vi "UI Initialize.vi"(8 "error in (no error)":errorcluster, 11 "TestEngine in":refnum<class "TestEngine.lvclass">) -> (0 "error out":errorcluster, 3 "TestEngine out":refnum<class "TestEngine.lvclass">)   [LabVIEW 2019, in "TestEngine.lvlib" / "TestEngine.lvclass"]
uses:
  TestEngine.lvclass
  C:/Program Files (x86)/National Instruments/LabVIEW 2019/vi.lib/NI/Event Source Actor/Event Source/Event Source/Event Source.lvclass
  TestEngineReference.lvclass
  C:/Program Files (x86)/National Instruments/LabVIEW 2019/vi.lib/NI/Event Source Actor/Event Source/Event/Event.lvclass
  <vilib>/NI/Event Source Actor/Event Source/Event/Event.lvclass/Event.ctl
  TestEngine.lvclass/TestEngine.ctl
  <vilib>/NI/Event Source Actor/Event Source/Event/Event.lvclass
  <vilib>/NI/Event Source Actor/Event Source/Event Source/Event Source.lvclass
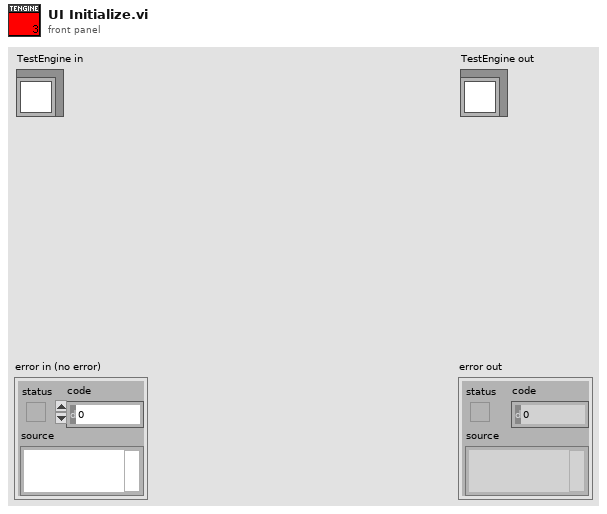
[diagram p1: front panel]
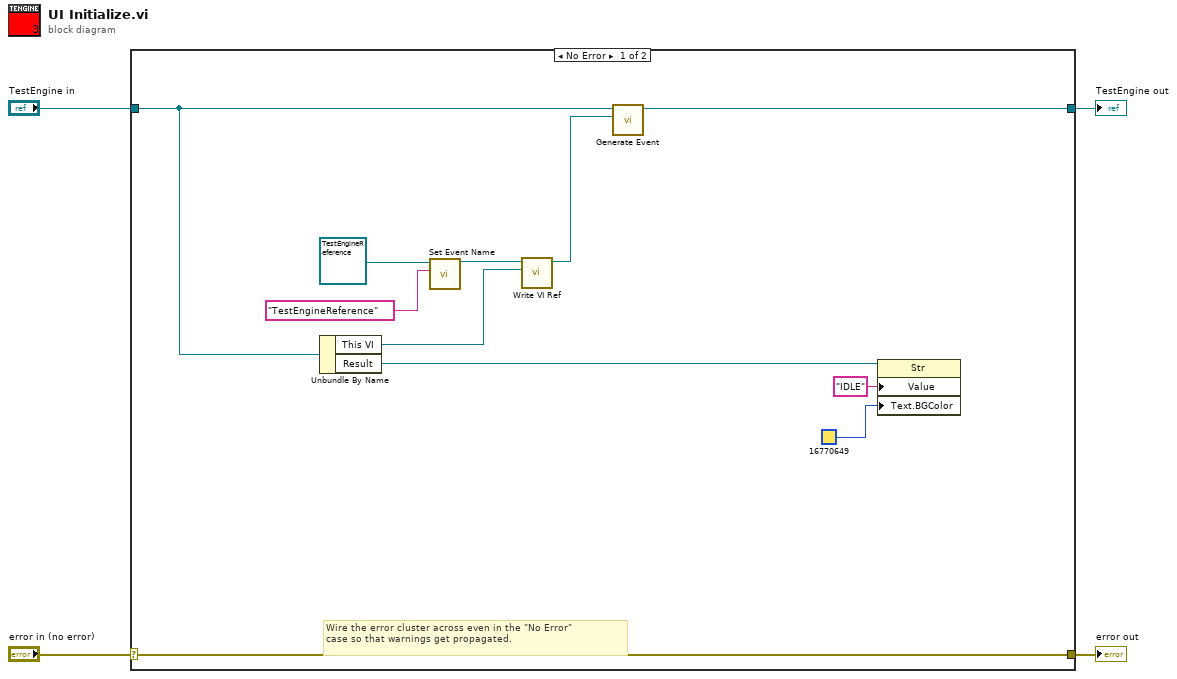
[diagram p0: block diagram]
diagram:
  n1 = case shown="No Error" "error in (no error)" {
    selector: "error in (no error)" -> [w15 w17]
    tunnel: [w15 w17] -> w3
    tunnel: [w8 w16] -> w1
    tunnel: "TestEngine in" -> [w9 w16]
    frame No Error {
      # "Wire the error cluster across even in the \"No Error\"\ncase so that warnings get propagated."
      n2 = Unbundle By Name(w9) -> ("This VI"=w10:refnum<vi>, "Result"=w7:refnum<vi>)
      n3 = call <vilib>:"Set Event Name.vi"("Name (Generic)"="TestEngineReference", "Event In"=refnum<class "TestEngineReference.lvclass"> refnum ("TestEngine.lvlib:TestEngineReference.lvclass")) -> ("Event Out"=w12:refnum<class "TestEngineReference.lvclass">)  [unwired: 9 in]
      n4 = call-dynamic "Write VI Ref.vi"("VI Ref"=w10, "TestEngineReference in"=w12) -> ("TestEngineReference out"=w11:refnum<class "TestEngineReference.lvclass">)  [unwired: 8 in, 1 out]
      n5 = call <vilib>:"Generate Event.vi"("Event"=w11, "Event Source In"=w9) -> ("Event Source Out"=w8:refnum<class "TestEngine.lvclass">)  [unwired: 8 in, 1 out]
      n6 = property class="Str"(reference=w7, "Value"="IDLE", "Text.BGColor"=u32 16770649 ("Text.Text Colors:BG Color")) -> ()  [unwired: 1 in, 2 out]
    }
    frame Error {
    }
  }
  "error out" <- w3
  "TestEngine out" <- w1
